vi "Acoustic Properties Project Output SubVI.vi"(0 "Stimiulation Duration":dbl=10.0, 3 "Upper Frequency":u32, 4 "Speaker Device ID":u32) -> ()   [LabVIEW 2018]
uses:
  <vilib>/sound2/lvsound2.llb/Sampling Mode.ctl
  <vilib>/sound2/lvsound2.llb/Sound Data Format.ctl
  <vilib>/sound2/lvsound2.llb/Sound Output Set Volume (Single).vi
  <vilib>/sound2/lvsound2.llb/Sound Output Write (DBL Single).vi
panel:
  in  "Volume":dbl=40.0
  out "Generated Sound":waveform(dbl)(graph)
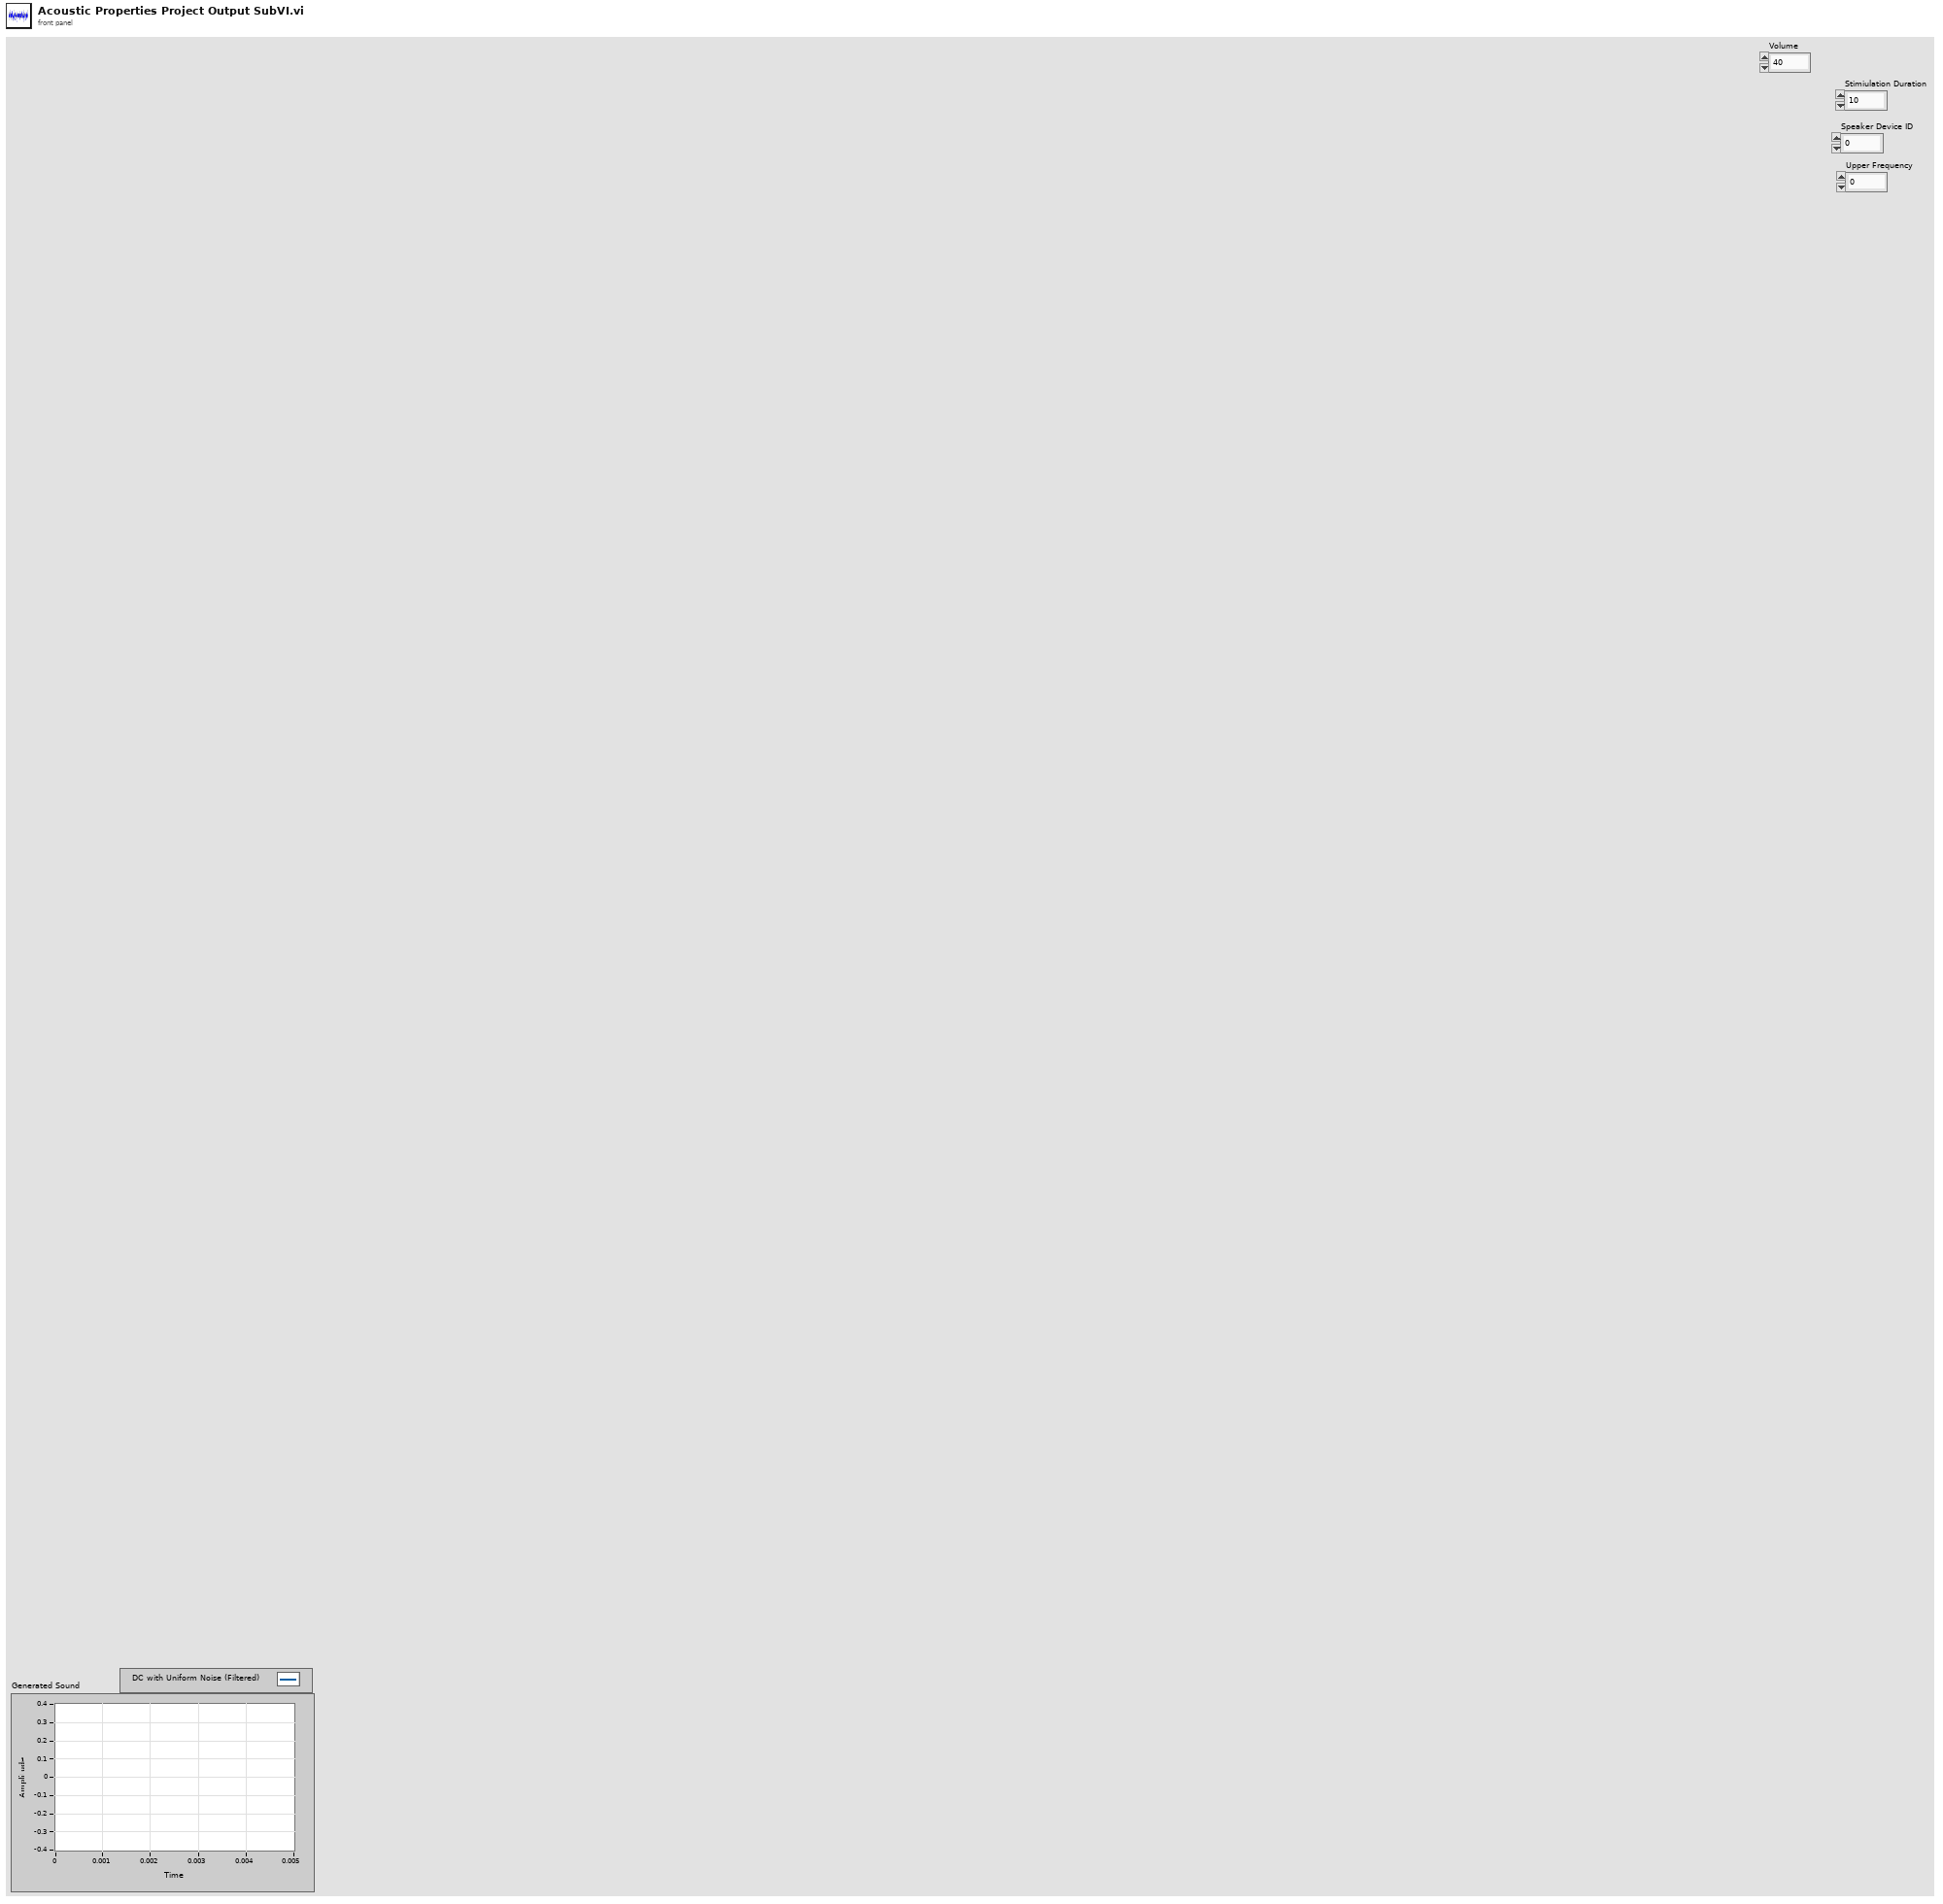
[diagram p1: front panel]
types:
  T1 = typedef "Sound Data Format.ctl" = cluster{"sample rate (S/s)":dbl, "number of channels":i32, "bits per sample":i32}
  T2 = typedef "Sampling Mode.ctl" = i32
  T3 = typedef "Sound Output Task ID.ctl" = u32
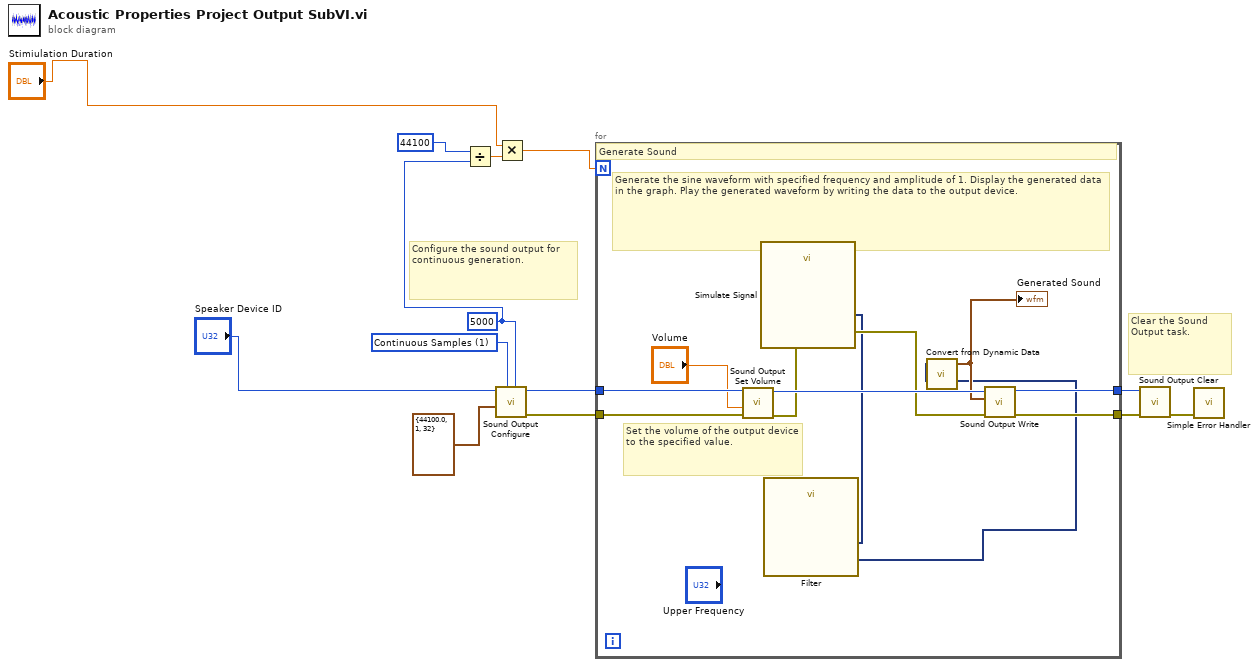
[diagram p0: block diagram]
diagram:
  w6 = 5000 ("Number of Samples/ch")
  w9 = T2 1 items=["Finite Samples", "Continuous Samples"] ("sample mode")
  # "Configure the sound output for continuous generation."
  # "Clear the Sound Output task."
  n1 = Divide(x=44100, y=w6) -> (x/y=w4:dbl)
  n2 = call <vilib>:"Sound Output Configure.vi"("number of samples/ch"=w6, "sample mode"=w9, "sound format"=T1 {"sample rate (S/s)"=44100.0, "number of channels"=1, "bits per sample"=32} ("Sound Format"), "device ID"="Speaker Device ID") -> ("error out"=w13:errorcluster, "task ID"=w12:T3)  [unwired: 6 in]
  n3 = Multiply(x="Stimiulation Duration", y=w4) -> (x*y=w2:dbl)
  n4 = for {
    N: w2 -> [_]
    tunnel: w12 -> [w21]
    tunnel: [w24] -> w10
    tunnel: w13 -> [w23]
    tunnel: [w19] -> w11
    # "Set the volume of the output device to the specified value."
    # "Generate the sine waveform with specified frequency and amplitude of 1. Display the generated data in the graph. Play the generated waveform by writing the data to the output device."
    # "Generate Sound"
    n5 = call-poly <vilib>:"Sound Output Set Volume.vi"("error in (no error)"=w23, "volume"="Volume", "task ID"=w21) -> ("error out"=w17:errorcluster, "task ID out"=w22:T3)  [unwired: 7 in]
    n6 = call "Simulate Signal"("error in (no error)"=w17) -> ("DC with Uniform Noise"=w15:dynamicdata, "error out"=w16:errorcluster)  [unwired: 13 in]
    n7 = call "Filter"("Signal"=w15) -> ("Filtered Signal"=w14:dynamicdata)  [unwired: 9 in, 1 out]
    n8 = call "Convert from Dynamic Data"("Dynamic Data Type"=w14) -> ("Waveform"=w18:waveform(dbl))  [unwired: 3 in]
    "Generated Sound" <- w18
    n9 = call-poly <vilib>:"Sound Output Write.vi"("error in (no error)"=w16, "data"=w18, "task ID"=w22) -> ("error out"=w19:errorcluster, "task ID out"=w24:T3)  [unwired: 7 in]
  }
  n10 = call <vilib>:"Sound Output Clear.vi"("error in (no error)"=w11, "task ID"=w10) -> ("error out"=w8:errorcluster)  [unwired: 9 in]
  n11 = call <vilib>:"Simple Error Handler.vi"("error in (no error)"=w8) -> ()  [unwired: 4 in, 5 out]
